vi "Main.vi"(8 "error in":errorcluster, 11 "TCP Send in":refnum<class "TCP Send.lvclass">) -> (0 "error out":errorcluster, 3 "TCP Send out":refnum<class "TCP Send.lvclass">)   [LabVIEW 2020, in "TCP Send.lvclass"]
doc: "The Queued Message Handler of a Worker."
uses:
  TCP Send.lvclass
  C:/Program Files (x86)/National Instruments/LabVIEW 2020/vi.lib/addons/_Workers/Library/Classes/Worker/Worker.lvclass
  Initialization Data.ctl
  <vilib>/addons/_Workers/Library/Classes/Message Queue/Message Queue.lvclass
  TCP Send.lvclass/TCP Send.ctl
  <vilib>/addons/_Workers/Library/Classes/EHL/EHL.lvclass
  <vilib>/addons/_Workers/Library/Classes/Worker/Worker.lvclass
  <vilib>/addons/_Workers/Library/Classes/Error Handler/Error Handler.lvclass
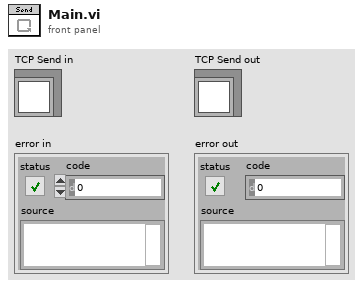
[diagram p1: front panel]
types:
  T1 = typedef "TCP Send.lvclass/Initialization Data.ctl" = cluster{"String":string, "connection ID":refnum<k5>, "End Point":refnum<class "Message Queue.lvclass">}
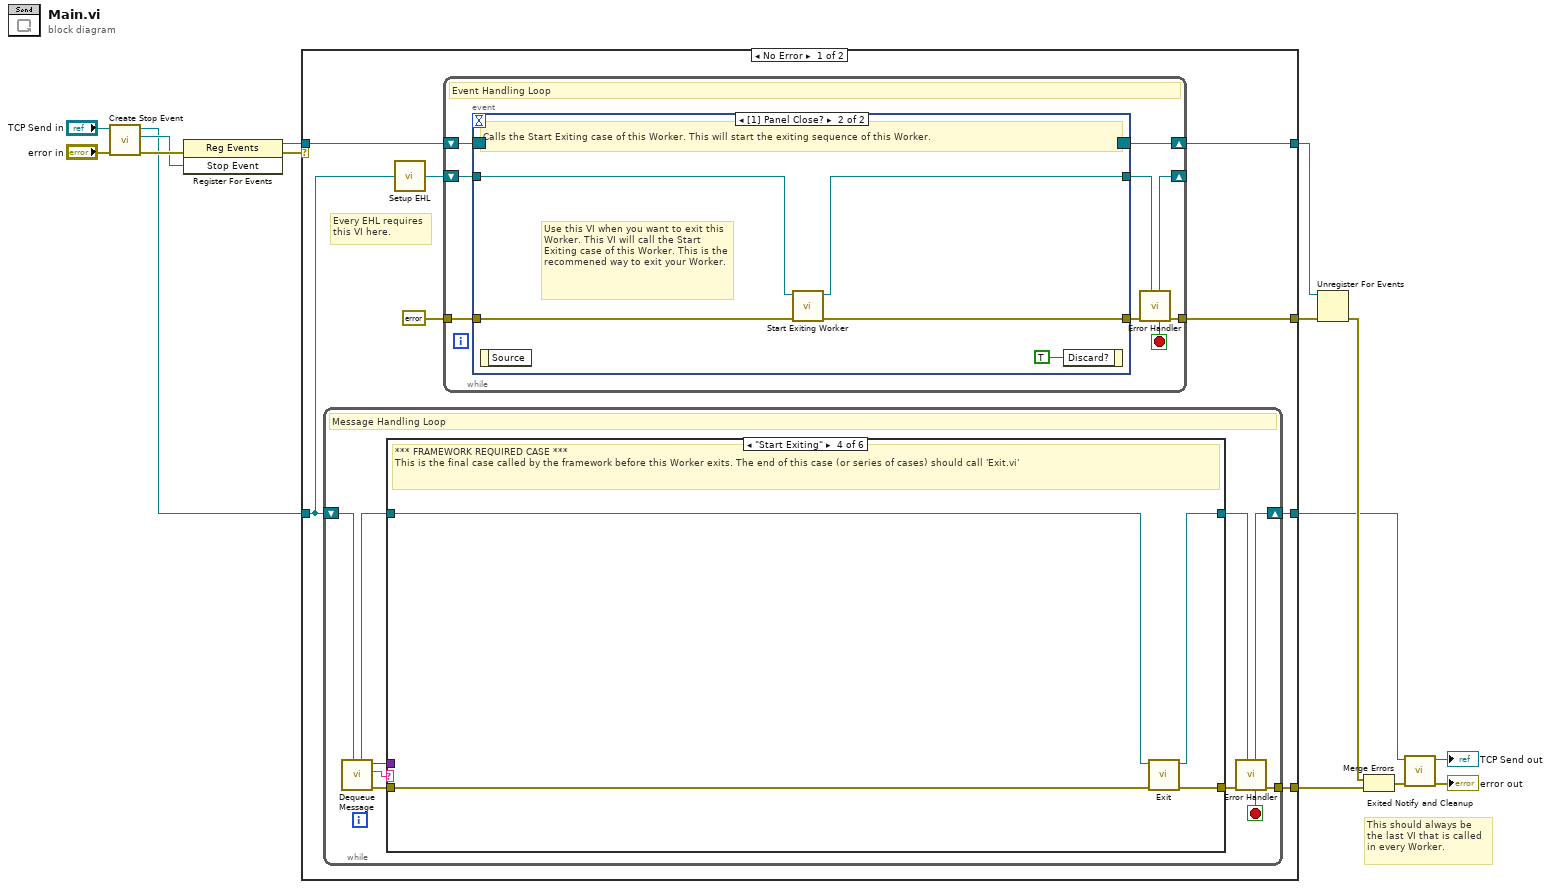
[diagram p0: block diagram]
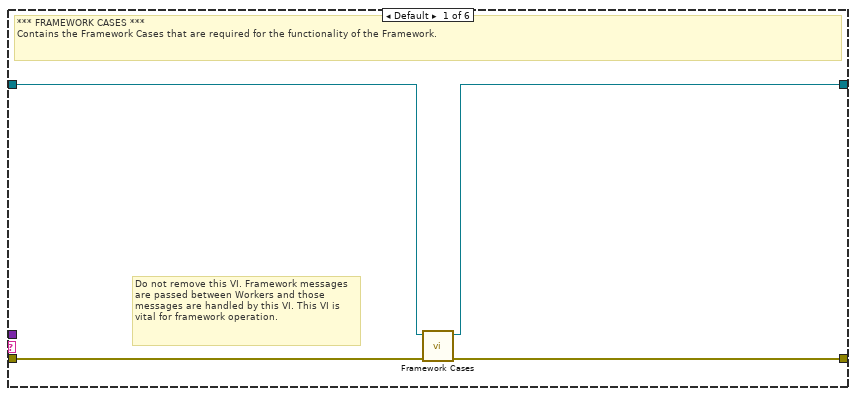
[diagram p2: hidden frame]
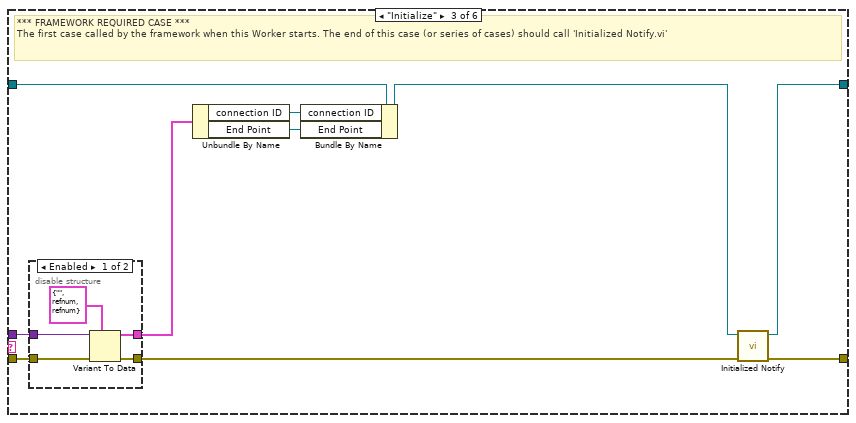
[diagram p4: hidden frame]
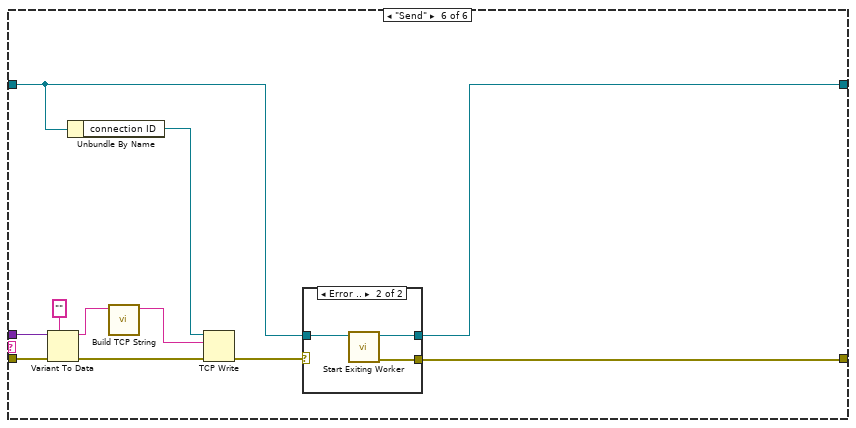
[diagram p7: hidden frame]
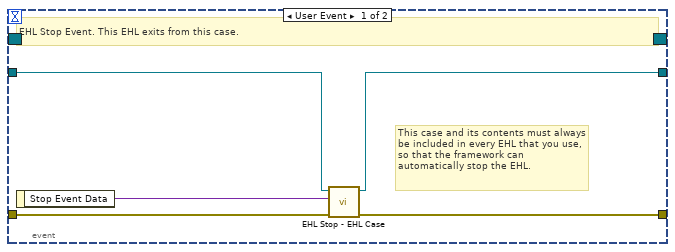
[diagram p9: hidden frame]
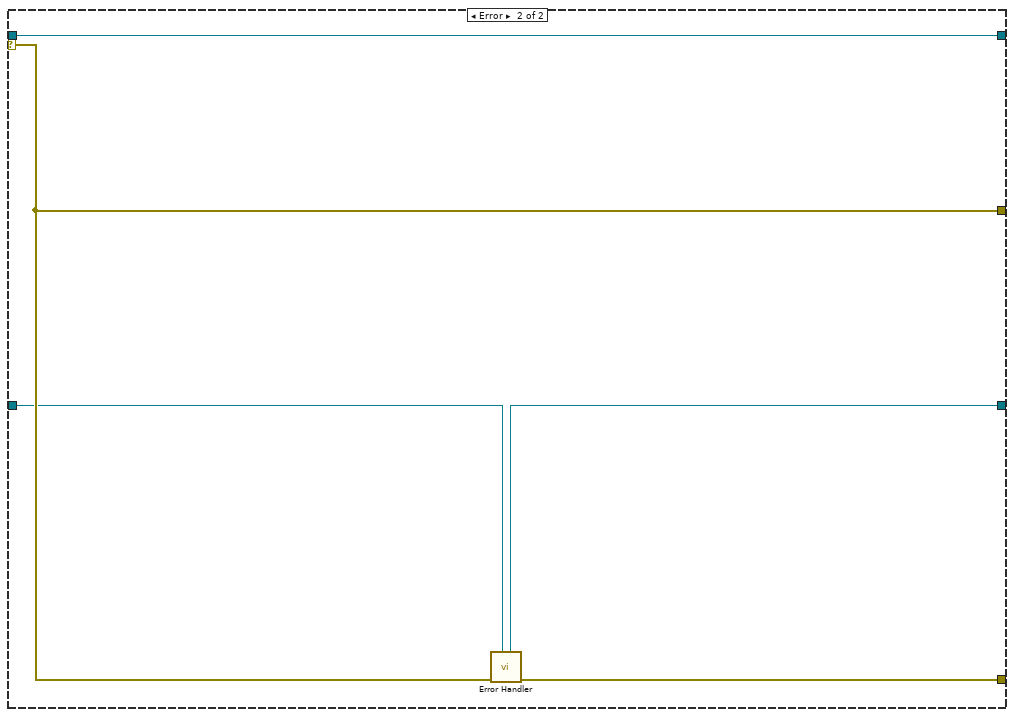
[diagram p10: hidden frame]
diagram:
  # "This should always be the last VI that is called in every Worker."
  n1 = call <vilib>:"Create Stop Event.vi"("error in"="error in", "Worker"="TCP Send in") -> ("error out"=w10:errorcluster, "Stop Event"=w7:refnum<user-event>, "Worker out"=w4:refnum<class "TCP Send.lvclass">)  [unwired: 7 in]
  n2 = register-events(error in=w10, w7) -> (reference out=w9:refnum<event-registration>, error out=w1:errorcluster)  [unwired: 1 in]
  n3 = case shown="No Error" w1 {
    tunnel: w4 -> [w18 w98]
    tunnel: [w16 w99] -> w8
    tunnel: w9 -> [w23 w100]
    tunnel: [w20 w101] -> w14
    tunnel: [w22 w100] -> w13
    tunnel: [w17 w97] -> w11
    selector: w1 -> [_ w101]
    frame No Error {
      # "Every EHL requires\nthis VI here."
      n4 = while {
        shift-right: [w31] -> w17
        shift-left: w18 -> [w33]
        tunnel: [w32] -> w16
        stop <- w24 stop-if-true
        # "Message Handling Loop"
        n5 = call <vilib>:"Dequeue Message.vi"("Worker"=w33) -> ("error out"=w30:errorcluster, "Case out"=w25:string, "Data out"=w26:variant, "Worker out"=w28:refnum<class "TCP Send.lvclass">)  [unwired: 6 in, 1 out]
        n6 = case "WORKERS MHL Case Structure (DO NOT CHANGE LABEL NAME)" shown="\"Start Exiting\"" w25 {
          tunnel: w30 -> [w37 w38 w47 w56 w60 w72]
          tunnel: [w36 w38 w49 w59 w60 w64] -> w29
          tunnel: w28 -> [w35 w39 w46 w57 w61 w63]
          tunnel: [w34 w39 w48 w58 w61 w62] -> w27
          tunnel: w26 -> [_ _ w44 _ _ w70]
          frame Default {
            # "Do not remove this VI. Framework messages are passed between Workers and those messages are handled by this VI. This VI is vital for framework operation."
            # "*** FRAMEWORK CASES ***\nContains the Framework Cases that are required for the functionality of the Framework."
            n7 = call <vilib>:"Framework Cases.vi"("error in"=w37, "Worker"=w35) -> ("error out"=w36:errorcluster, "Worker out"=w34:refnum<class "TCP Send.lvclass">)  [unwired: 8 in]
          }
          frame "------ FRAMEWORK REQUIRED CASES ------" {
            # "Start of Framework Required Cases"
          }
          frame "Initialize" {
            # "*** FRAMEWORK REQUIRED CASE ***\nThe first case called by the framework when this Worker starts. The end of this case (or series of cases) should call 'Initialized Notify.vi'"
            n8 = disable-structure shown="Enabled" {
              disable-tunnel: w47 -> [w54 w55]
              disable-tunnel: [w53 w55] -> w45
              disable-tunnel: w44 -> [w52 _]
              disable-tunnel: [w50 _] -> w42
              frame Enabled {
                n9 = Variant To Data(error in=w54, type=T1 {"String"="", "connection ID"=refnum, "End Point"=refnum} ("Initialization Data"), Variant=w52) -> (data=w50:T1, error out=w53:errorcluster)
              }
              frame Disabled {
              }
            }
            n10 = Unbundle By Name(w42) -> ("connection ID"=w41:refnum<k5>, "End Point"=w40:refnum<class "Message Queue.lvclass">)
            n11 = Bundle By Name(cluster=w46, "connection ID"=w41, "End Point"=w40) -> (w43:refnum<class "TCP Send.lvclass">)
            n12 = call <vilib>:"Initialized Notify.vi"("error in"=w45, "Worker"=w43) -> ("error out"=w49:errorcluster, "dup Worker out"=w48:refnum<class "TCP Send.lvclass">)  [unwired: 8 in]
          }
          frame "Start Exiting" {
            # "*** FRAMEWORK REQUIRED CASE ***\nThis is the final case called by the framework before this Worker exits. The end of this case (or series of cases) should call 'Exit.vi'"
            n13 = call <vilib>:"Exit.vi"("error_in"=w56, "Worker"=w57) -> ("error out"=w59:errorcluster, "dup Worker out"=w58:refnum<class "TCP Send.lvclass">)  [unwired: 8 in]
          }
          frame "-----------------------------------------------" {
            # "End of Framework Required Cases"
          }
          frame "Send" {
            n14 = Variant To Data(error in=w72, type="", Variant=w70) -> (data=w67:string, error out=w71:errorcluster)
            n15 = Unbundle By Name(w63) -> ("connection ID"=w68:refnum<k5>)
            n16 = call "Build TCP String.vi"("Data"=w67) -> ("TCP String"=w66:string)  [unwired: 10 in]
            n17 = TCP Write(connection ID=w68, data in=w66, error in (no error)=w71) -> (error out=w65:errorcluster)  [unwired: 1 in, 2 out]
            n18 = case shown="Error .." w65 {
              selector: w65 -> [w74 _]
              tunnel: [w74 w77] -> w64
              tunnel: w63 -> [w73 w76]
              tunnel: [w73 w75] -> w62
              frame No Error {
              }
              frame Error {
                n19 = call <vilib>:"Start Exiting Worker.vi"("Worker"=w76) -> ("error out"=w77:errorcluster, "dup Worker out"=w75:refnum<class "TCP Send.lvclass">)  [unwired: 9 in]
              }
            }
          }
        }
        n20 = call <vilib>:"Error Handler.vi"("Worker"=w27, "error_in"=w29) -> ("error out"=w32:errorcluster, "Stop Loop"=w24:bool, "Worker out"=w31:refnum<class "TCP Send.lvclass">)  [unwired: 7 in]
      }
      n21 = call <vilib>:"Setup EHL.vi"("Worker"=w18) -> ("Worker out"=w19:refnum<class "TCP Send.lvclass">)  [unwired: 14 in]
      n22 = while "Event Handling Loop" {
        shift-right: [w86] -> w22
        shift-left: w23 -> [w85]
        tunnel: [w81] -> w20
        tunnel: errorcluster {"status"=FALSE, "code"=0, "source"=""} ("error constant") -> [w83]
        shift-right: [w79] -> _
        shift-left: w19 -> [w84]
        stop <- w78 stop-if-true
        # "Event Handling Loop"
        n23 = event shown="[1] Panel Close?" {
          selector: w85 -> [_ _]
          dyn-events: [_ _] -> w86
          timeout: _ -> [_ _]
          tunnel: [w90 w95] -> w82
          tunnel: w83 -> [w91 w94]
          tunnel: w84 -> [w89 w93]
          tunnel: [w88 w92] -> w80
          event User Event {
            # "This case and its contents must always be included in every EHL that you use, so that the framework can automatically stop the EHL."
            # "EHL Stop Event. This EHL exits from this case."
            n24 = event-data() -> ("Stop Event Data"=w87:variant)  [unwired: 1 in]
            n25 = call <vilib>:"EHL Stop - EHL Case.vi"("error in"=w91, "Stop Event Data"=w87, "Worker"=w89) -> ("error out"=w90:errorcluster, "Worker out"=w88:refnum<class "TCP Send.lvclass">)  [unwired: 7 in]
          }
          event Panel Close? {
            # "Use this VI when you want to exit this Worker. This VI will call the Start Exiting case of this Worker. This is the recommened way to exit your Worker."
            # "Calls the Start Exiting case of this Worker. This will start the exiting sequence of this Worker."
            n26 = event-data() -> ()  [unwired: 1 in, 1 out]
            n27 = call <vilib>:"Start Exiting Worker.vi"("error in"=w94, "Worker"=w93) -> ("error out"=w95:errorcluster, "dup Worker out"=w92:refnum<class "TCP Send.lvclass">)  [unwired: 8 in]
            n28 = event-data("Discard?"=TRUE) -> ()  [unwired: 1 in, 1 out]
          }
        }
        n29 = call <vilib>:"Error Handler.vi"("Worker"=w80, "error_in"=w82) -> ("error out"=w81:errorcluster, "Stop Loop"=w78:bool, "Worker out"=w79:refnum<class "TCP Send.lvclass">)  [unwired: 7 in]
      }
    }
    frame Error {
      n30 = call <vilib>:"Error Handler.vi"("Worker"=w98, "error_in"=w101) -> ("error out"=w99:errorcluster, "Worker out"=w97:refnum<class "TCP Send.lvclass">)  [unwired: 7 in, 1 out]
    }
  }
  n31 = Unregister For Events(event registration refnum=w13, error in=w14) -> (error out=w15:errorcluster)
  n32 = Merge Errors(w15, w8) -> (w12:errorcluster)
  n33 = call <vilib>:"Exited Notify and Cleanup.vi"("error_in"=w12, "Worker"=w11) -> ("error out"=→"error out":errorcluster, "dup Worker out"=→"TCP Send out":refnum<class "TCP Send.lvclass">)  [unwired: 8 in]
